vi "SQLite Insert TestSequence.vi"(6 "UpdateAlarm?":bool, 7 "Main":string="0", 8 "error in (no error)":errorcluster, 9 "Sequence Value":T1, 10 "SequenceNum":string, 11 "Items":string) -> (0 "error out":errorcluster, 2 "Update SQL":string, 3 "Insert DB String":string)   [LabVIEW 2017, in "SQLite.lvclass"]
doc: "保存校准的结果值,.\n2015-11-03 16:29:50\nBy：蒋松\nEmail：jiangsong@outlook.com\nSina: @sushu1051"
uses:
  SQLite.lvclass
  SQLiteFileName.ctl
  TabelFullName.ctl
  <vilib>/Utility/error.llb/Trim Whitespace.vi
  <userlib>/LabSQL/LabSQL.lvlib
  <userlib>/sushu/sushu.lvlib
panel:
  # "insert 之前要先backup原有的数据，使Items在对应条目的最大值+1\n2015-11-03 16:45:40\nBy：蒋松\nEmail：jiangsong@outlook.com\nSina: @sushu1051"
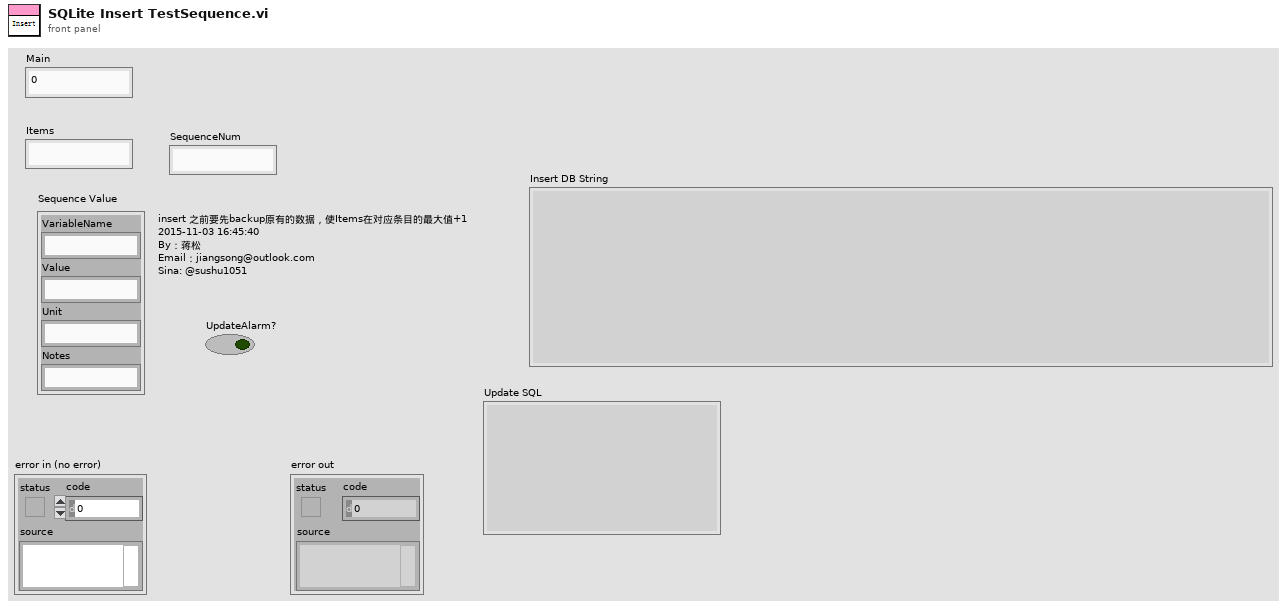
[diagram p1: front panel]
types:
  T1 = cluster{"VariableName":string, "Value":string, "Unit":string, "Notes":string}
  T2 = typedef "SQLite.lvclass/TabelFullName.ctl" = string
  T3 = typedef "SQLite.lvclass/SQLiteFileName.ctl" = string
  T4 = enum32{"invalid app kind", "Development System", "Run Time System", "Student Edition", "Embedded LabVIEW", "Evaluation", "Custom"}
  T5 = enum32{"Invalid", "Standard", "Closed", "Hidden", "Minimized", "Maximized"}
  T6 = enum16{"Other", "SQL2008", "SQLite", "Access", "MySQL"}
  T7 = cluster{"Core":cluster{"Current VI Reference":refnum<vi>, "Close Panel on Exit?":bool}}
  T8 = cluster{"Current VI Reference":refnum<vi>, "Close Panel on Exit?":bool}
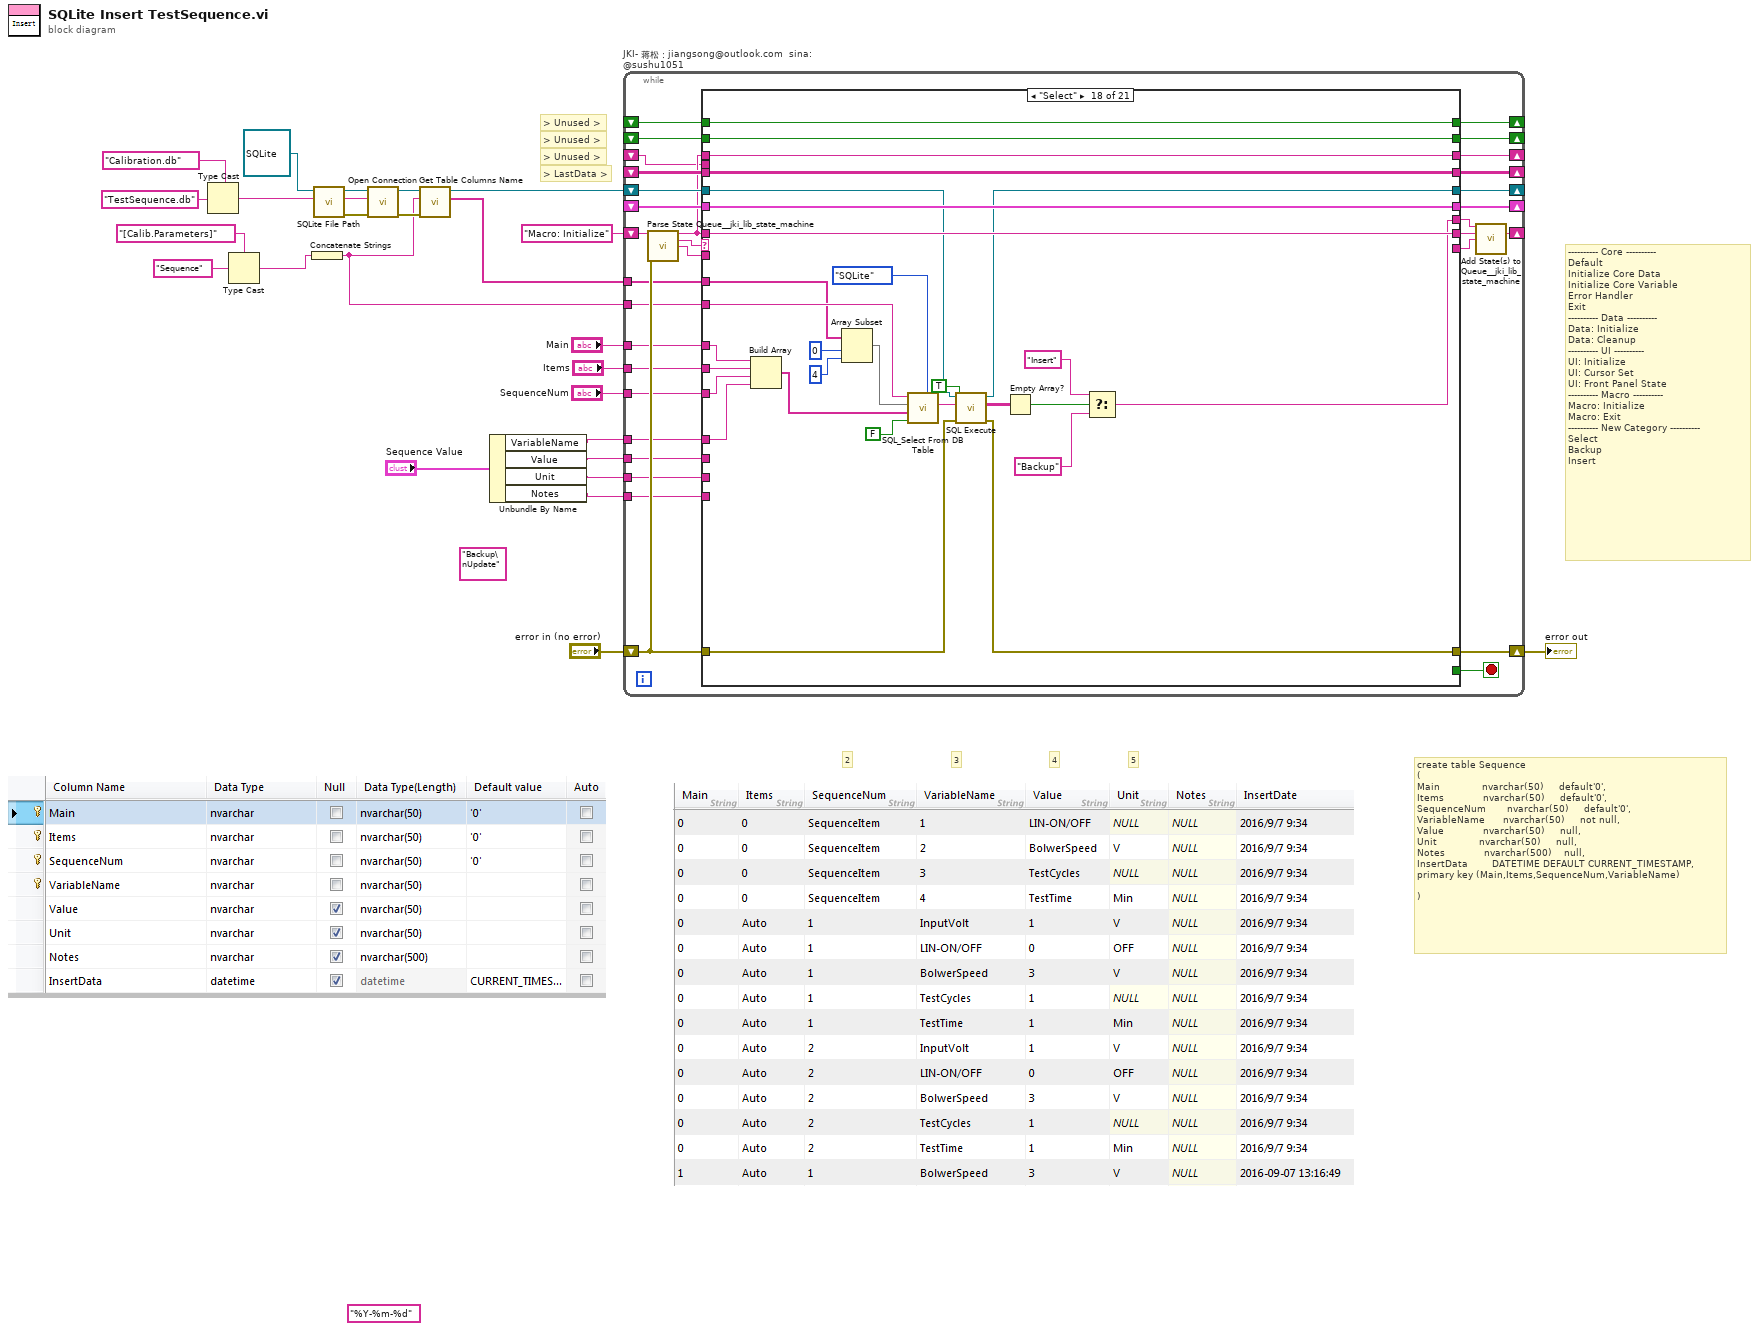
[diagram p0: block diagram]
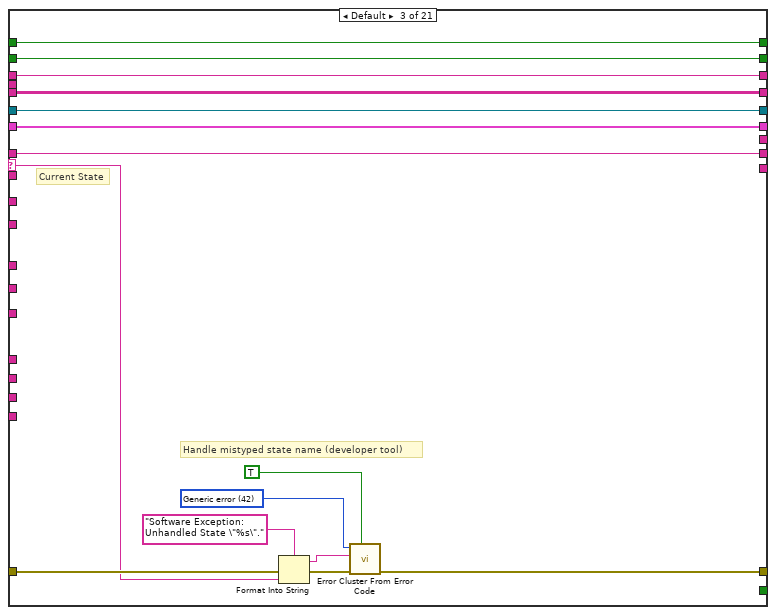
[diagram p4: hidden frame]
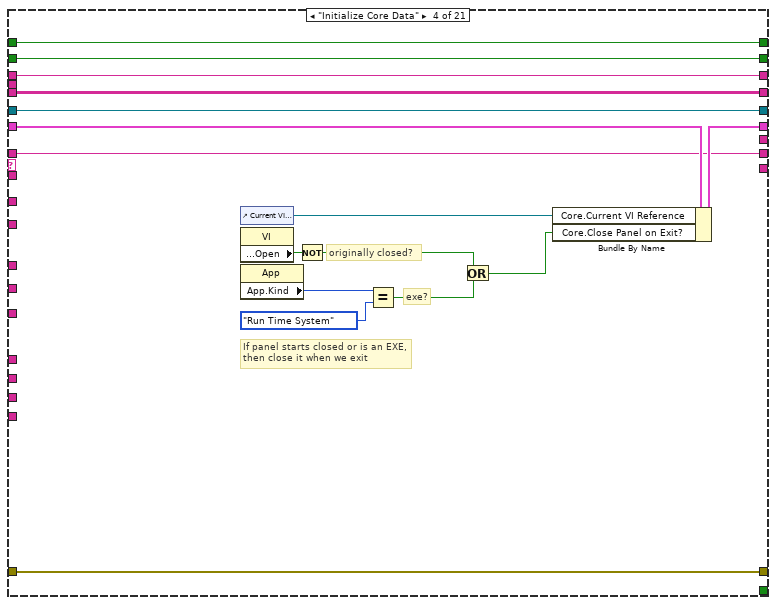
[diagram p5: hidden frame]
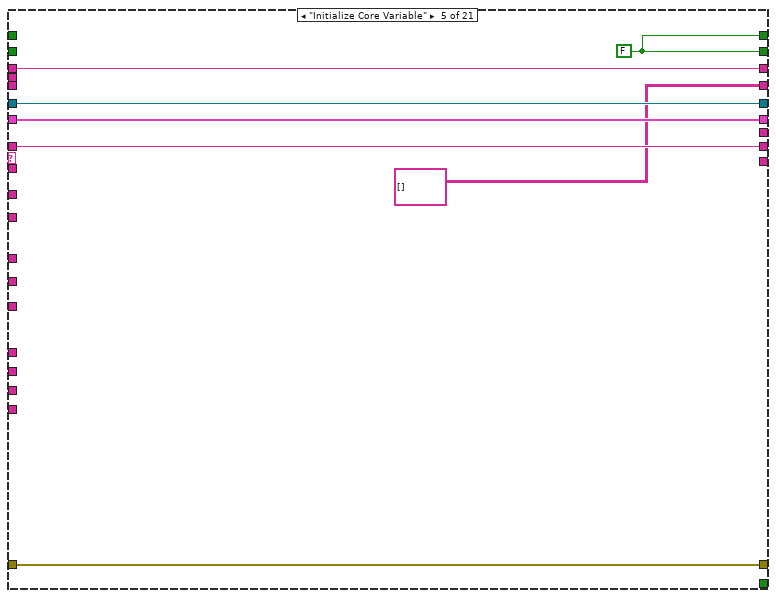
[diagram p6: hidden frame]
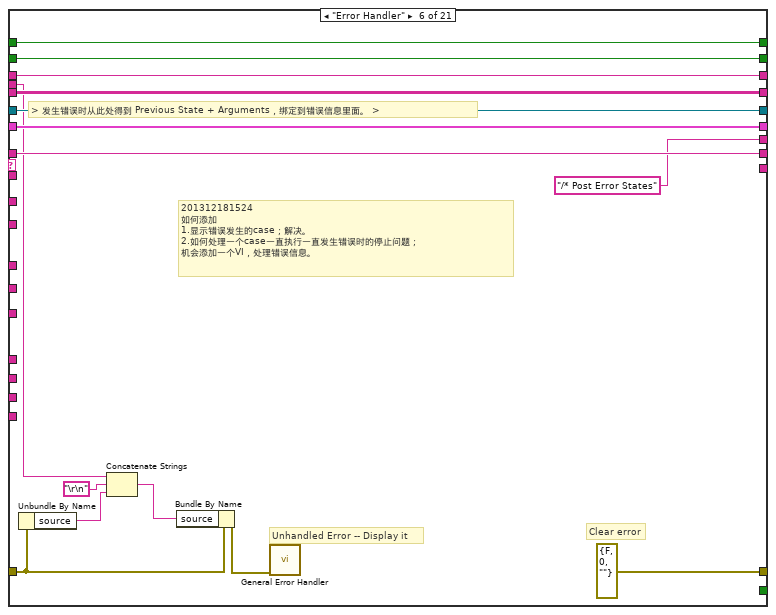
[diagram p7: hidden frame]
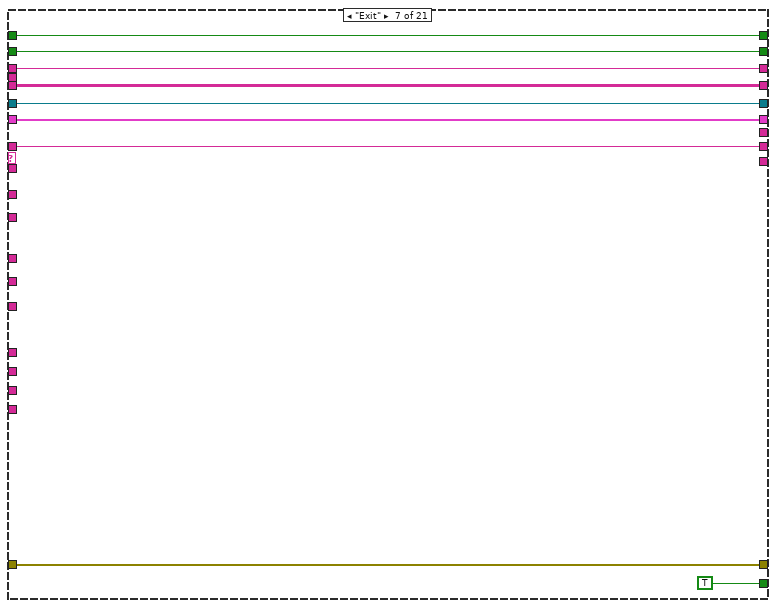
[diagram p8: hidden frame]
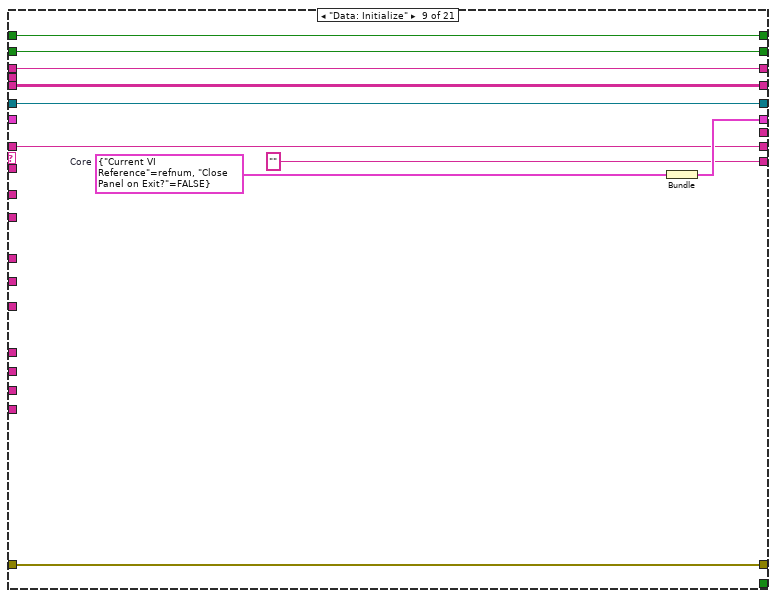
[diagram p10: hidden frame]
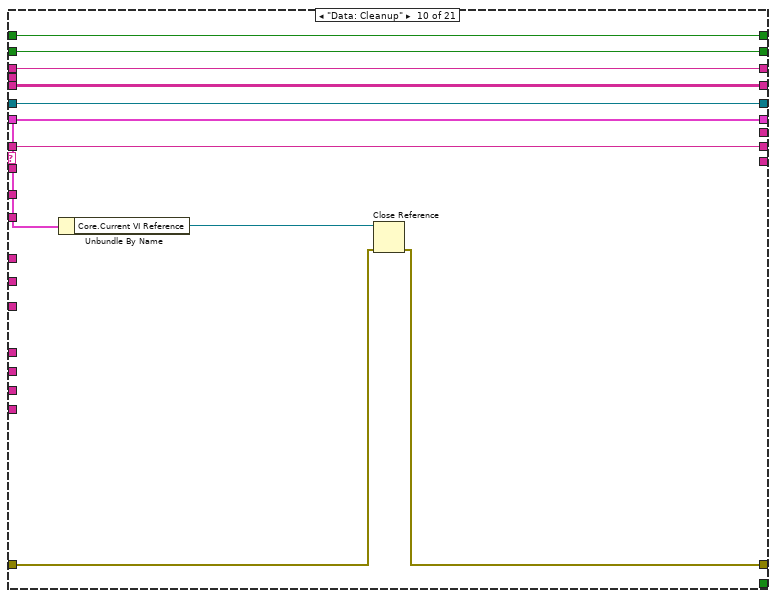
[diagram p11: hidden frame]
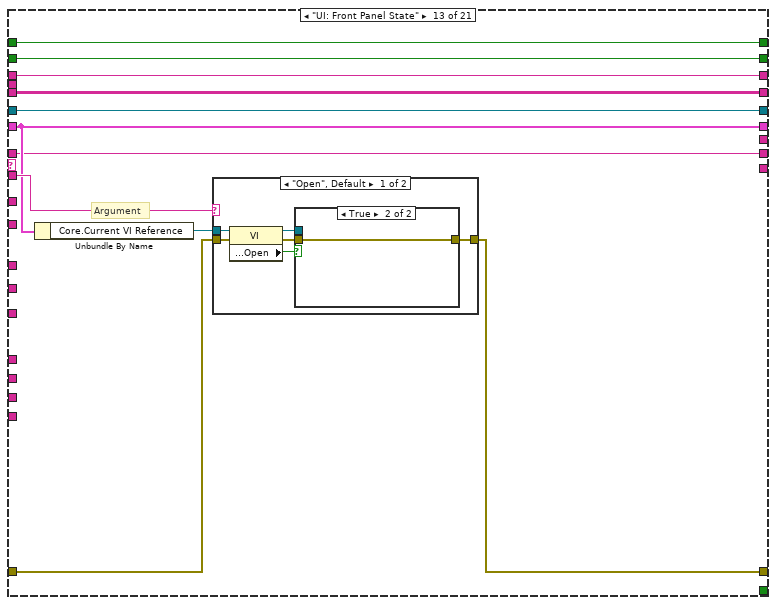
[diagram p14: hidden frame]
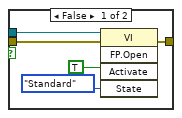
[diagram p15: hidden frame]
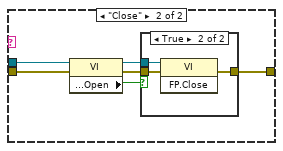
[diagram p16: hidden frame]
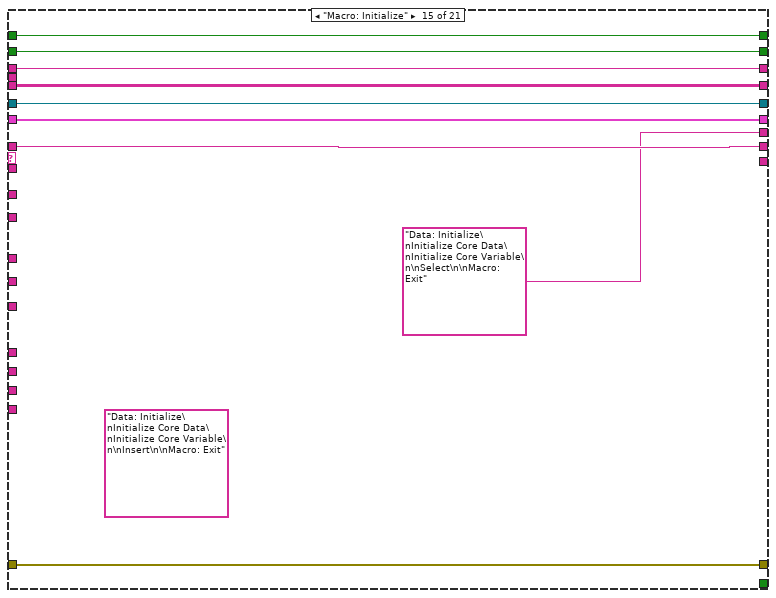
[diagram p19: hidden frame]
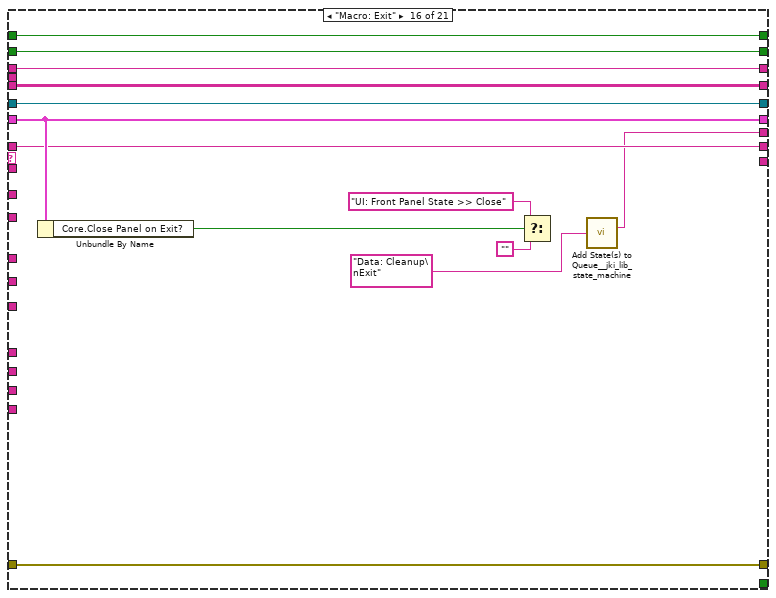
[diagram p20: hidden frame]
diagram:
  (unwired) "Backup\nUpdate" ("Select SQL CMD")
  (unwired) "%Y-%m-%d" ("time format string (%c)")
  # "create table Sequence\n(\nMain              nvarchar(50)     default'0',\nItems             nvarchar(50)     default'0',\nSequenceNum       nvarchar(50)     default'0',\nVariableName      nvarchar(50)     not null,\nValue             nvarchar(50)     null,\nUnit              nvarchar(50)     null,\nNotes             nvarchar(500)    null,\nInsertData        DATETIME DEFAULT CURRENT_TIMESTAMP,\nprimary key (Main,Items,SequenceNum,VariableName)\n\n)"
  # "5"
  # "4"
  # "3"
  # "2"
  # "> Unused >"
  # "> LastData >"
  # "> Unused >"
  # "> Unused >"
  # "---------- Core ----------\nDefault\nInitialize Core Data\nInitialize Core Variable\nError Handler\nExit\n---------- Data ----------\nData: Initialize\nData: Cleanup\n---------- UI ----------\nUI: Initialize\nUI: Cursor Set\nUI: Front Panel State\n---------- Macro ----------\nMacro: Initialize\nMacro: Exit\n---------- New Category ----------\nSelect\nBackup\nInsert"
  n1 = Type Cast(type=T3 "Calibration.db" ("SQLiteFileName"), x="TestSequence.db" ("Remaining States")) -> (*(type *) &x=w12:T3)
  n2 = Type Cast(type=T2 "[Calib.Parameters]" ("TabelFullName"), x="Sequence" ("Remaining States")) -> (*(type *) &x=w15:T2)
  n3 = Concatenate Strings(w15) -> (w1:string)
  n4 = call "SQLite File Path.vi"("SQLiteFileName"=w12, "SQLite in"=refnum<class "SQLite.lvclass"> refnum ("SQLite.lvclass")) -> ("error out"=w9:errorcluster, "string"=w6:string, "SQLite out"=w8:refnum<class "SQLite.lvclass">)  [unwired: 7 in]
  n5 = call-dynamic "Open Connection.vi"("error in (no error)"=w9, "ConnectionString"=w6, "HostDB in"=w8) -> ("error out"=w5:errorcluster, "HostDB out"=w4:refnum<class "SQLite.lvclass">)  [unwired: 7 in]
  n6 = call-dynamic "Get Table Columns Name.vi"("error in (no error)"=w5, "TableName"=w1, "HostDB in"=w4) -> ("ColunmsList"=w2:string[], "HostDB out"=w3:refnum<class "SQLite.lvclass">)  [unwired: 4 in, 3 out]
  n7 = Unbundle By Name("Sequence Value") -> ("VariableName"=w20:string, "Value"=w19:string, "Unit"=w18:string, "Notes"=w17:string)
  n8 = while "JKI- 蒋松：jiangsong@outlook.com  sina: @sushu1051" {
    shift-right: [w56] -> w24
    shift-left: "error in (no error)" -> [w54]
    shift-right: [w44] -> _
    shift-left: "Macro: Initialize" -> [w45]
    shift-right: [w51] -> _
    shift-left: _ -> [w27]
    shift-right: [w52] -> _
    shift-left: _ -> [w53]
    shift-right: [w46] -> _
    shift-left: _ -> [w49]
    shift-right: [w47] -> _
    shift-left: w3 -> [w40]
    shift-right: [w48] -> _
    shift-left: _ -> [w50]
    shift-right: [w39] -> _
    shift-left: _ -> [w38]
    tunnel: w2 -> [w37]
    tunnel: w1 -> [w36]
    tunnel: "Main" -> [w35]
    tunnel: "Items" -> [w34]
    tunnel: w20 -> [w33]
    tunnel: w19 -> [w32]
    tunnel: w18 -> [w31]
    tunnel: w17 -> [w30]
    tunnel: "SequenceNum" -> [w29]
    stop <- w55 stop-if-true
    n9 = call <vilib>:"Parse State Queue__jki_lib_state_machine.vi"("State Queue"=w45, "Error In (no error)"=w54) -> ("Remaining States"=w28:string, "Current State"=w58:string, "Arguments"=w57:string)  [unwired: 10 in, 1 out]
    n10 = case shown="\"Select\"" w58 {
      selector: w58 -> [_ _ w77 _ _ _ _ _ _ _ _ _ _ _ _ _ _ _ _ _ _]
      tunnel: w28 -> [w66 w68 w76 w91 w110 w117 w129 w138 w147 w156 w166 w174 w182 w215 w224 w233 w245 w276 w291 w328 w362]
      tunnel: w57 -> [_ _ _ _ _ _ _ _ _ _ _ _ w185 _ _ _ _ _ _ _ _]
      tunnel: [w65 w74 w78 w102 w112 errorcluster {"status"=FALSE, "code"=0, "source"=""} ("error out") w131 w140 w151 w158 w168 w176 w186 w217 w226 w240 w248 w254 w286 w304 w331] -> w56
      tunnel: w54 -> [w65 w74 w79 w102 w112 w121 w131 w140 w151 w159 w168 w176 w187 w217 w226 w240 w248 w255 w287 w305 w333]
      tunnel: [w66 w68 w76 w91 w110 w117 w129 w138 w147 w156 w166 w174 w182 w215 w224 w233 w245 w276 w291 w328 w362] -> w43
      tunnel: [_ _ _ _ _ _ TRUE _ _ _ _ _ _ _ _ _ _ _ _ _ _] -> w55
      tunnel: w53 -> [w64 w73 w89 w105 _ w127 w136 w144 w154 w164 w172 w180 w191 w221 w230 w243 w251 w280 w294 w327 w361]
      tunnel: w28 -> [w63 w72 w88 w104 w106 w126 w135 w143 w153 w163 w171 w179 w190 w220 w229 w242 w250 w279 w293 w326 w360]
      tunnel: [w64 w73 w89 w105 w109 w127 w136 w144 w154 w164 w172 w180 w191 w221 w230 w243 w251 w280 w294 w327 w361] -> w52
      tunnel: [w63 w72 w88 w104 w106 w126 w135 w143 w153 w163 w171 w179 w190 w220 w229 w242 w250 w279 w293 w326 w360] -> w51
      tunnel: w50 -> [w62 w71 w87 w103 _ w125 w134 w142 w152 w162 w170 w178 w189 w219 w228 w241 w249 w278 w289 w325 w359]
      tunnel: w40 -> [w60 w69 w86 w92 w108 w115 w130 w139 w148 w157 w167 w175 w183 w216 w225 w234 w246 w259 w288 w309 w335]
      tunnel: w49 -> [w61 w70 w85 w94 w111 w124 w133 w141 _ w160 w169 w177 w184 w218 w227 w235 w247 w277 w292 w324 w358]
      tunnel: [w62 w71 w87 w103 string[][] [] ("Result Set") w125 w134 w142 w152 w162 w170 w178 w189 w219 w228 w241 w249 w278 w289 w325 w359] -> w48
      tunnel: [w60 w69 w86 w92 w108 w115 w130 w139 w148 w157 w167 w175 w183 w216 w225 w234 w246 w258 w288 w306 w336] -> w47
      tunnel: [w61 w70 w85 w93 w111 w124 w133 w141 w149 w160 w169 w177 w184 w218 w227 w235 w247 w277 w292 w324 w358] -> w46
      tunnel: [_ _ _ _ _ "/* Post Error States" _ _ _ _ _ _ _ _ "Data: Initialize\nInitialize Core Data\nInitialize Core Variable\n\nSelect\n\nMacro: Exit" w232 _ w261 w284 _ _] -> w42
      tunnel: [_ _ _ _ _ _ _ _ "" _ _ _ _ _ _ _ _ _ _ _ _] -> w41
      tunnel: w38 -> [w59 w67 w75 w90 _ w114 w128 w137 w145 w155 w165 w173 w181 w214 w222 w231 w244 w275 w290 w323 w357]
      tunnel: [w59 w67 w75 w90 w109 w114 w128 w137 w145 w155 w165 w173 w181 w214 w222 w231 w244 w275 w290 w323 w357] -> w39
      tunnel: w37 -> [_ _ _ _ _ _ _ _ _ _ _ _ _ _ _ _ _ w268 _ w317 w342]
      tunnel: w36 -> [_ _ _ _ _ _ _ _ _ _ _ _ _ _ _ _ _ w274 _ w318 w347]
      tunnel: w35 -> [_ _ _ _ _ _ _ _ _ _ _ _ _ _ _ _ _ w273 _ w316 w354]
      tunnel: w34 -> [_ _ _ _ _ _ _ _ _ _ _ _ _ _ _ _ _ w272 _ w315 w353]
      tunnel: w33 -> [_ _ _ _ _ _ _ _ _ _ _ _ _ _ _ _ _ w270 _ w314 w352]
      tunnel: w32 -> [_ _ _ _ _ _ _ _ _ _ _ _ _ _ _ _ _ _ _ w313 w350]
      tunnel: w31 -> [_ _ _ _ _ _ _ _ _ _ _ _ _ _ _ _ _ _ _ w312 w349]
      tunnel: w30 -> [_ _ _ _ _ _ _ _ _ _ _ _ _ _ _ _ _ _ _ w311 w348]
      tunnel: w29 -> [_ _ _ _ _ _ _ _ _ _ _ _ _ _ _ _ _ w271 _ w310 w351]
      tunnel: w27 -> [_ _ _ _ _ w113 _ _ _ _ _ _ _ _ _ _ _ _ _ _ _]
      frame "", "Idle" {
      }
      frame "---------- Core ----------" {
      }
      frame Default {
        w81 = 42 items=["No error", "Argument error", "Memory is full", "Out of zone", "End of file", "File already open", "Generic file I/O error", "File not found", "File permission error", "Disk is full", "Duplicate path", "Too many files open", "System feature not enabled", "Resource file not found", "Cannot add resource", "Resource not found", "Image not found", "Image memory error", "Pen does not exist", "Config type invalid", "Config token not found", "Config parse error", "Config memory error", "Bad external code format", "Bad external code offset", "External code not present", "Null window", "Destroy window error", "Null menu", "Print aborted", "Bad print record", "Print driver error", "Windows error during printing", "Memory error during printing", "Print dialog error", "Generic print error", "Invalid device refnum", "Device not found", "Device parameter error", "Device unit error", "Cannot open device", "Device call aborted", "Generic error", "Cancelled by user", "Object ID too low", "Object ID too high", "Object not in heap", "Unknown heap", "Unknown object (invalid DefProc)", "Unknown object (DefProc not in table)", "Message out of range", "Invalid (null) method", "Unknown message", "Manager call not supported", "Bad address", "Network operation in progress", "Network operation timed out", "Connection is busy", "Network attribute not supported", "Network error", "Address in use", "System out of memory", "Connection aborted", "Connection refused", "Not connected", "Already connected", "Connection closed", "Initialization error (interapplication manager)", "Bad occurrence", "Wait on unbound occurrence handler", "Occurrence queue overflow", "Datalog type conflict", "Unused", "Unrecognized type (interapplication manager)", "Memory corrupt", "Failed to make temporary DLL", "Old CIN version", "Drag socket not found", "Failed to load drop-object", "Failed to register OLE object", "Failed to release OLE object", "Format specifier type mismatch", "Unknown format specifier", "Too few format specifiers", "Too many format specifiers", "Scan failed", "Newer CIN version", "Error converting to variant", "Runtime menu error", "Password tampered", "Variant attribute not found", "Incompatible variant data type", "Event data is not available", "Event Store is not present", "Occurrence is not found", "Event Queue is not created", "Event info is not available", "Refnum passed is NULL", "Error retrieving Class GUID", "Error retrieving CoClass GUID", "Error retrieving TypeLib GUID.", "Bad built application magic bytes.", "Specific driver is different from the specific driver associated with the Logical Name.", "There is no session opened to the class driver.", "Max Error", "MAX - Error with config objects", "MAX - Error loading configuration", "MAX - Group not supported"]
        # "Current State"
        # "Handle mistyped state name (developer tool)"
        n11 = Format Into String(format string="Software Exception: Unhandled State \"%s\"." ("message"), error in=w79, w77) -> (resulting string=w82:string, error out=w83:errorcluster)  [unwired: 1 in]
        n12 = call <vilib>:"Error Cluster From Error Code.vi"("show call chain? (False)"=TRUE, "error in (no error)"=w83, "error message (\"\")"=w82, "error code (0)"=w81) -> ("error out"=w78:errorcluster)  [unwired: 5 in]
      }
      frame "Initialize Core Data" {
        # "originally closed?"
        # "exe?"
        # "If panel starts closed or is an EXE, then close it when we exit"
        n13 = control-ref of="Current VI Reference"() -> (w101:refnum<vi>)
        n14 = property class="VI"() -> ("Front Panel.Open"=w95:bool)  [unwired: 2 in, 2 out]
        n15 = property class="App"() -> ("App.Kind"=w96:T4)  [unwired: 2 in, 2 out]
        n16 = Not(x=w95) -> (.not. x?=w98:bool)
        n17 = Equal?(x=w96, y=T4."Run Time System" ("Application:Kind")) -> (x = y?=w99:bool)
        n18 = Or(x=w98, y=w99) -> (x .or. y?=w100:bool)
        n19 = Bundle By Name(cluster=w94, "Core.Current VI Reference"=w101, "Core.Close Panel on Exit?"=w100) -> (w93:T7)
      }
      frame "Initialize Core Variable" {
        w109 = FALSE
      }
      frame "Error Handler" {
        # "> 发生错误时从此处得到 Previous State + Arguments，绑定到错误信息里面。 >"
        # "201312181524\n如何添加\n1.显示错误发生的case；解决。\n2.如何处理一个case一直执行一直发生错误时的停止问题；\n机会添加一个VI，处理错误信息。"
        # "Clear error"
        # "Unhandled Error -- Display it"
        n20 = Unbundle By Name(w121) -> ("source"=w119:string)
        n21 = Concatenate Strings(w113, "\r\n", w119) -> (w118:string)
        n22 = Bundle By Name(cluster=w121, "source"=w118) -> (w122:errorcluster)
        n23 = call <vilib>:"General Error Handler.vi"("error in (no error)"=w122) -> ()  [unwired: 10 in, 5 out]
      }
      frame "Exit" {
      }
      frame "---------- Data ----------" {
      }
      frame "Data: Initialize" {
        w150 = T8 {"Current VI Reference"=refnum, "Close Panel on Exit?"=FALSE}  # Core
        n24 = Bundle("Core"=w150) -> (w149:T7)  [unwired: 1 in]
      }
      frame "Data: Cleanup" {
        n25 = Unbundle By Name(w160) -> ("Core.Current VI Reference"=w161:refnum<vi>)
        n26 = Close Reference(reference=w161, error in (no error)=w159) -> (error out=w158:errorcluster)
      }
      frame "---------- UI ----------" {
      }
      frame "UI: Initialize" {
      }
      frame "UI: Front Panel State" {
        # "Argument"
        n27 = Unbundle By Name(w184) -> ("Core.Current VI Reference"=w188:refnum<vi>)
        n28 = case shown="\"Open\", Default" w185 {
          tunnel: w187 -> [w195 w208]
          tunnel: [w197 w209] -> w186
          tunnel: w188 -> [w196 w206]
          frame "Open", Default {
            n29 = property class="VI"(reference=w196, error in=w195) -> (reference out=w193:refnum<vi>, error out=w194:errorcluster, "Front Panel.Open"=w192:bool)
            n30 = case shown="True" w192 {
              tunnel: [w200 w203] -> w197
              tunnel: w194 -> [w199 w203]
              tunnel: w193 -> [w198 _]
              frame False {
                n31 = invoke class="VI" method="FP.Open"(reference=w198, error in=w199, "Activate"=TRUE, "State"=T5."Standard") -> (error out=w200:errorcluster)  [unwired: 1 in, 4 out]
              }
              frame True {
              }
            }
          }
          frame "Close" {
            n32 = property class="VI"(reference=w206, error in=w208) -> (reference out=w205:refnum<vi>, error out=w207:errorcluster, "Front Panel.Open"=w204:bool)
            n33 = case shown="True" w204 {
              tunnel: [w210 w213] -> w209
              tunnel: w207 -> [w210 w212]
              tunnel: w205 -> [_ w211]
              frame False {
              }
              frame True {
                n34 = invoke class="VI" method="FP.Close"(reference=w211, error in=w212) -> (error out=w213:errorcluster)  [unwired: 1 in, 2 out]
              }
            }
          }
        }
      }
      frame "---------- Macro ----------" {
      }
      frame "Macro: Initialize" {
        (unwired) "Data: Initialize\nInitialize Core Data\nInitialize Core Variable\n\nInsert\n\nMacro: Exit"
      }
      frame "Macro: Exit" {
        n35 = Unbundle By Name(w235) -> ("Core.Close Panel on Exit?"=w236:bool)
        n36 = Select(t="UI: Front Panel State >> Close", s=w236, f="") -> ()  [unwired: 1 out]
        n37 = call <vilib>:"Add State(s) to Queue__jki_lib_state_machine.vi"("State(s) at Back (\"\")"="Data: Cleanup\nExit") -> ("States Out"=w232:string)  [unwired: 14 in]
      }
      frame "---------- New Category ----------" {
      }
      frame "Select" {
        n38 = Build Array(w273, w272, w271, w270) -> (w269:string[])
        n39 = Array Subset(array=w268, index=0, length=4) -> (w265:string[])
        n40 = call <userlib>:"SQL_Select From DB Table.vi"("DB Type"=T6."SQLite", "Check ASCII?"=FALSE, "ColumnsValue"=w269, "ColumnsNameList"=w265, "TableName"=w274) -> ("Select SQL CMD"=w256:string)  [unwired: 6 in]
        n41 = call-dynamic "SQL Execute.vi"("error in (no error)"=w255, "Return Data (T)"=TRUE, "Command Text"=w256, "HostDB in"=w259) -> ("error out"=w254:errorcluster, "Table Control"=w257:string[][], "HostDB out"=w258:refnum<class "SQLite.lvclass">)  [unwired: 3 in, 2 out]
        n42 = Empty Array?(array=w257) -> (empty?=w264:bool)
        n43 = Select(t="Insert" ("Select SQL CMD"), s=w264, f="Backup" ("Select SQL CMD")) -> (s? t:f=w261:string)
      }
      frame "Backup" {
        n44 = case shown="True" "UpdateAlarm?" {
          tunnel: w287 -> [w296 w299]
          tunnel: [w296 w298] -> w286
          tunnel: [TRUE ("OK?") w297] -> w285
          frame False {
          }
          frame True {
            n45 = call <userlib>:"Errors Handle Dialoge.vi"("error in (no error)"=w299, "Message"="Before Insert you should Backup old TestSequence data.\nDo you want update?") -> ("error out"=w298:errorcluster, "OK?"=w297:bool)  [unwired: 8 in]
          }
        }
        n46 = Select(t="Update" ("Select SQL CMD"), s=w285, f="") -> (s? t:f=w284:string)
      }
      frame "Insert" {
        n47 = Build Array(w316, w315, w310, w314, w313, w312, w311) -> (w319:string[])
        n48 = Array Subset(array=w317, index=0, length=7) -> (w322:string[])
        n49 = call <userlib>:"SQL_Insert DB Table.vi"("DB Type"=enum16{"Other", "SQL2008", "SQLite"}."SQLite", "ColumnsValue"=w319, "ColumnsName"=w322, "Table Name"=w318) -> ("Insert DB String"=w308:string)  [unwired: 7 in]
        "Insert DB String" <- w308
        n50 = call-dynamic "SQL Execute.vi"("error in (no error)"=w305, "Return Data (T)"=FALSE, "Command Text"=w308, "HostDB in"=w309) -> ("error out"=w303:errorcluster, "HostDB out"=w307:refnum<class "SQLite.lvclass">)  [unwired: 3 in, 3 out]
        n51 = call-dynamic "Close Connection.vi"("error in (no error)"=w303, "HostDB in"=w307) -> ("error out"=w304:errorcluster, "HostDB out"=w306:refnum<class "SQLite.lvclass">)  [unwired: 8 in]
      }
      frame "Update" {
        n52 = Build Array(w350, w349, w348) -> (w346:string[])
        n53 = Build Array(w354, w353, w351, w352) -> (w345:string[])
        n54 = Array Subset(array=w342, index=0, length=4) -> (w339:string[])
        n55 = call <userlib>:"Build string_ColumnsName=ColumnsValue_Where and.vi"("DB Type"=T6."SQLite", "ColumnsValue"=w345, "Check ASCII?"=FALSE, "ColumnsNameList"=w339) -> ("ColumnName='ColumnValue'"=w344:string)  [unwired: 7 in]
        n56 = Array Subset(array=w342, index=4, length=3) -> (w343:string[])
        n57 = call <userlib>:"SQL_Update DB Table.vi"("where name='value'"=w344, "ColumnsValue"=w346, "ColumnsNameList"=w343, "TableName"=w347) -> ("Update CMD"=w334:string)  [unwired: 7 in]
        "Update SQL" <- w334
        n58 = call-dynamic "SQL Execute.vi"("error in (no error)"=w333, "Return Data (T)"=FALSE, "Command Text"=w334, "HostDB in"=w335) -> ("error out"=w332:errorcluster, "HostDB out"=w337:refnum<class "SQLite.lvclass">)  [unwired: 3 in, 3 out]
        n59 = call-dynamic "Close Connection.vi"("error in (no error)"=w332, "HostDB in"=w337) -> ("error out"=w331:errorcluster, "HostDB out"=w336:refnum<class "SQLite.lvclass">)  [unwired: 8 in]
      }
    }
    n60 = call <vilib>:"Add State(s) to Queue__jki_lib_state_machine.vi"("State(s) in Front (\"\")"=w42, "State(s) in (\"\")"=w43, "State(s) at Back (\"\")"=w41) -> ("States Out"=w44:string)  [unwired: 12 in]
  }
  "error out" <- w24
